vi "Sistema_2.vi"() -> ()   [LabVIEW 2017]
uses:
  <vilib>/Motion/Express/_s/nimc.ex.write.writeSetpoint.axis.vi
  <vilib>/Motion/Express/_s/nimc.fb.straightLineMove.startStraightLineMove.axis.modeAbsolute.0.vi
  <vilib>/Motion/Express/_s/nimc.fb.arcMove.startArcMove.coordinate.modeCircular.0.vi
  <vilib>/Motion/Express/_s/nimc.ex.read.readExecutionData.axis.vi
  <vilib>/Motion/BlockNode/FB.NIMotion.xnode
panel:
  in  "Array 2":T1(array[cluster])
  in  "Velocidad":dbl=10.0 format="%#_13g"
  out "x > y?":bool=TRUE
  out "done":bool=TRUE
  in  "Posición Inicial":cluster{"X":dbl, "Y":dbl, "Z":dbl}
  out "Paso":i32=69
  in  "Stop Button":bool
  out "EY":dbl(slide) scale=0.0..10.0
  out "EX":dbl(slide)=23.0 scale=0.0..10.0
  out "XY Graph":cluster{dbl[], dbl[]}(graph)={[0.0, 0.426423996, 1.426315789, 2.4263157890000002, 2.999891794, 3.0, 2.997709298, 2.215789474, 1.218080176, 1.0, 1.0, 1.0, 1.0, 1.0, 1.0, 0.45789473700000005, -0.0, -0.0, -0.0, -0.0, -0.0, -0.0, -0.0, 0.005048895, 0.32563547000000004, 1.194736842, 2.194736842, 2.894736842, 3.894736842, 4.894736842, 5.894736842, 6.727090094, 6.998255176, 7.0, 7.0, 7.0, 7.0, 7.0, 7.0, 7.0, 6.557894737, 6.0, 6.0, 6.0, 6.0, 6.0, 6.0, 5.557894737, 5.0, 5.0, 5.0, 5.0, 5.0, 5.0, 5.0, 4.157894737, 4.0, 4.0, 4.0, 4.0, 4.0, 4.0, 4.0, 4.048989208, 4.516094471, 5.436842105, 6.436842105, 7.436842105, 8.436842105, 9.436842105, 10.436842105, 11.387852897, 11.920747634, 12.0, 12.0, 11.916385042, 10.936842105, 10.5, 10.5, 10.5, 10.5, 10.5, 11.063157895, 11.979542936, 12.0, 12.0, 11.995418596, 11.529091619999999, 10.531578947, 9.531578947, 8.532151623, 8.002487327, 8.0, 8.0, 8.763157895, 9.5, 9.5, 9.5, 9.5, 9.5, 9.136842105, 8.066802093, 8.0, 8.0, 8.055501693, 8.564273623, 9.515789474, 10.515789474, 11.515789474, 12.515789474, 13.515789474, 14.514486319, 15.27534626, 15.499221793, 15.990506967, 16.0, 16.0, 15.584, 15.057894737, 14.5, 14.0, 14.116, 14.607617729, 15.601898554, 15.999811191, 16.0, 15.75, 15.105263158, 14.105263158, 13.5, 13.0, 13.0, 13.0, 13.0, 13.509032779, 14.486361958, 14.990506967, 15.0, 14.5, 13.836842105, 13.001629181, 13.0, 13.092082839, 13.707674496, 14.694736842, 15.694736842, 16.694736842, 17.694736842, 18.694736842, 19.602654003, 19.987062346000002, 20.0, 20.0, 20.0, 20.111486611, 21.084210526, 21.972723915, 22.0, 22.0, 21.415789474, 20.415789474, 20.0, 20.0, 20.111486611, 21.084210526, 21.972723915, 22.0, 22.0, 21.573576004, 20.573684211, 19.573684211, 19.0, 19.0, 19.0, 19.0, 19.0, 19.0, 19.0, 19.0, 19.167646748, 19.896481666, 20.894736842, 21.894736842, 22.894736842, 23.894736842, 24.994549846, 25.780379567, 25.999747518, 26.0, 26.0, 25.315789474, 24.218080176, 24.0, 24.0, 24.284282664, 25.284210526, 25.999927862, 26.0, 25.997709298, 25.215789474, 24.218080176, 24.0, 24.0, 24.284282664, 25.284210526, 25.999927862, 26.0, 25.99898191, 25.373684211, 24.373684211, 23.3747023, 23.0, 23.0, 23.0, 23.0, 23.0, 23.0, 23.0], [0.0, 0.0, 0.0, 0.0, 0.0, 0.5421052630000001, 1.0, 1.0, 1.0, 1.004581404, 1.568565328, 2.568421053, 3.568421053, 4.563839648, 4.999855725, 5.0, 5.0, 4.721283472, 3.789473684, 2.789473684, 1.6894736840000002, 0.689840197, 0.039900739000000005, 0.0, 0.0, 0.0, 0.0, 0.0, 0.0, 0.0, 0.0, 0.0, 0.0, 0.045163897, 0.71070666, 1.7105263160000002, 2.710526316, 3.610526316, 4.587072946, 4.997899781, 5.0, 5.0, 4.621142376, 3.631578947, 2.631578947, 1.532151623, 1.002487327, 1.0, 1.0, 1.3788576240000001, 2.268421053, 2.968421053, 3.868421053, 4.801204409, 5.0, 5.0, 4.97654663, 4.28929334, 3.289473684, 2.289473684, 1.289473684, 0.334637581, 0.000180344, 0.0, 0.0, 0.0, 0.0, 0.0, 0.0, 0.0, 0.0, 0.0, 0.0, 0.0, 0.742105263, 1.0, 1.0, 1.0, 1.5263157889999999, 2.526315789, 3.526315789, 4.0, 4.0, 4.0, 4.442105263, 5.0, 5.0, 5.0, 5.0, 5.0, 5.0, 5.0, 4.557894737, 4.0, 4.0, 4.0, 3.670425848, 2.6736842110000003, 1.673684211, 1.003258362, 1.0, 1.0, 0.657894737, -0.0, -0.0, -0.0, -0.0, -0.0, -0.0, -0.0, -0.0, -0.0, -0.0, -0.0, 0.490506967, 0.963157895, 1.933197907, 2.416, 2.5, 2.5, 3.025493033, 3.616, 4.0, 4.0, 4.249811191, 4.75, 5.0, 5.0, 5.0, 5.0, 4.5, 3.9157894740000003, 2.9157894740000003, 2.5, 2.0, 2.0, 1.509493033, 1.0, 0.5, 0.5, 0.5, 0.0, 0.0, 0.0, 0.0, 0.0, 0.0, 0.0, 0.0, 0.0, 0.0, 0.05435941800000001, 0.984210526, 1.929851108, 2.0, 2.0, 2.0, 2.342105263, 3.0, 3.0, 3.0, 3.0, 3.842105263, 4.0, 4.0, 4.0, 4.342105263, 5.0, 5.0, 5.0, 5.0, 5.0, 4.839704524, 3.989473684, 2.989473684, 1.989473684, 0.989473684, 0.14976916, -0.0, -0.0, -0.0, -0.0, -0.0, -0.0, -0.0, -0.0, -0.0, -0.0, 0.442105263, 1.0, 1.0, 1.0, 1.055743306, 1.986361958, 2.0, 2.0, 2.0, 2.542105263, 3.0, 3.0, 3.0, 3.055743306, 3.986361958, 4.0, 4.0, 4.0, 4.542105263, 5.0, 5.0, 5.0, 5.0, 5.0, 4.721283472, 3.789473684, 2.789473684, 1.789473684, 0.7894736840000001, 0.068190212]}
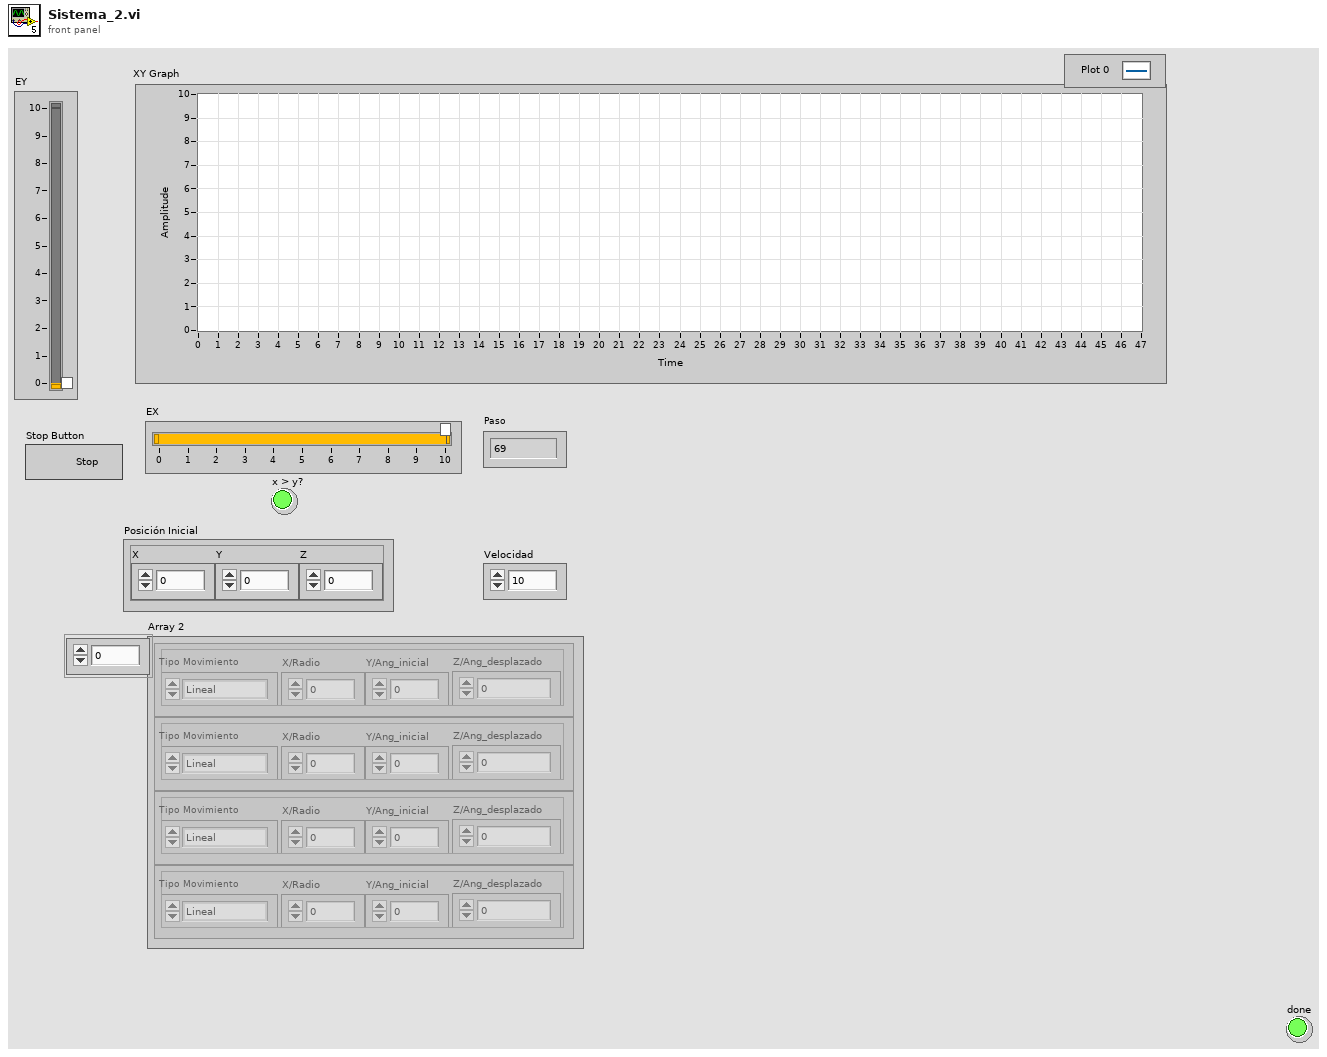
[diagram p1: front panel]
types:
  T1 = cluster{"Tipo Movimiento":enum16{"Lineal", "Circular"}, "X/Radio":dbl, "Y/Ang_inicial":dbl, "Z/Ang_desplazado":dbl}[]
  T2 = cluster{"Tipo Movimiento":enum16{"Lineal", "Circular"}, "X":dbl, "Y":dbl}[]
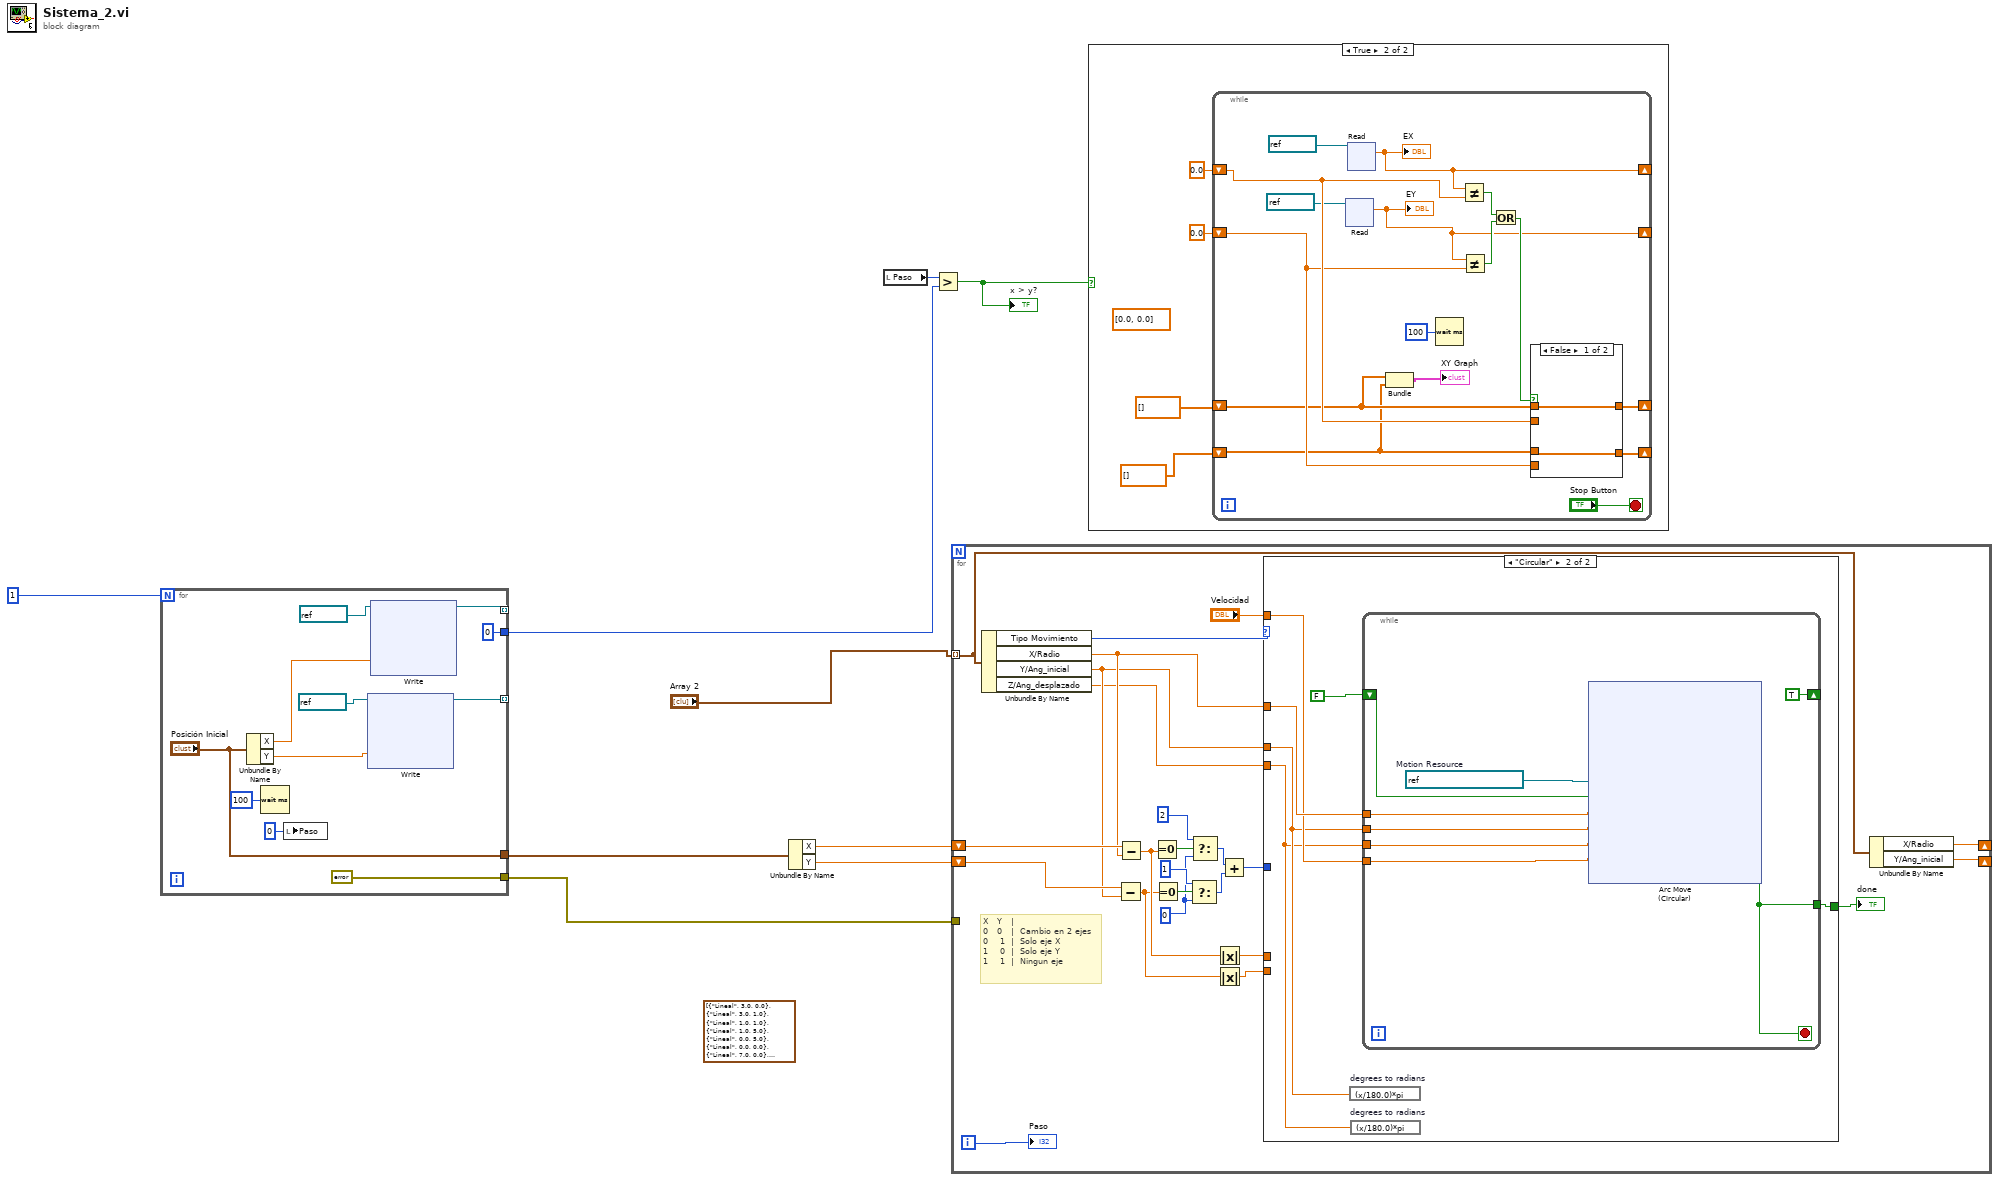
[diagram p0: block diagram]
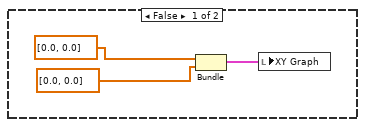
[diagram p2: hidden frame]
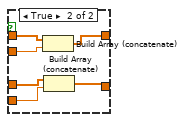
[diagram p3: hidden frame]
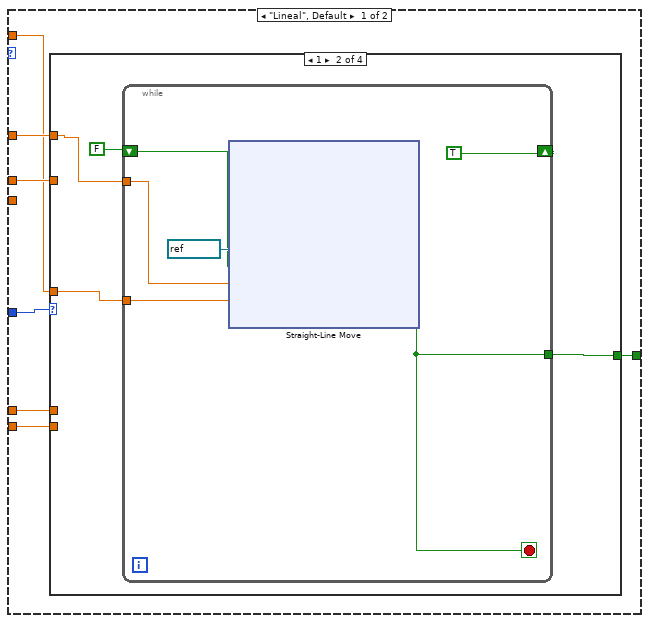
[diagram p4: hidden frame]
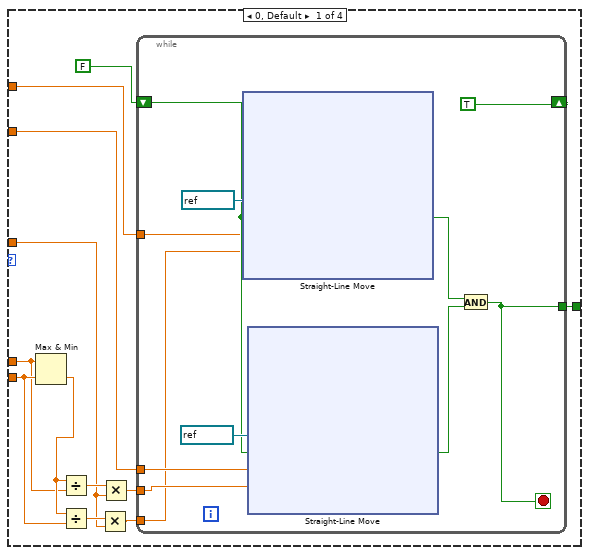
[diagram p5: hidden frame]
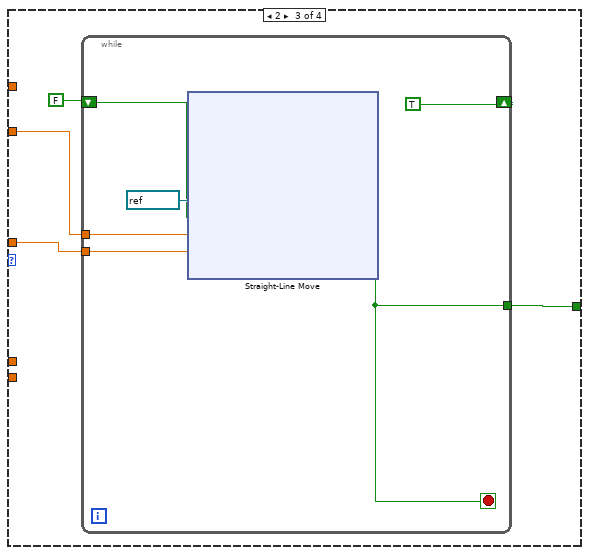
[diagram p6: hidden frame]
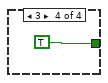
[diagram p7: hidden frame]
diagram:
  (unwired) T2 [{"Tipo Movimiento"=enum."Lineal", "X"=3.0, "Y"=0.0}, {"Tipo Movimiento"=enum."Lineal", "X"=3.0, "Y"=1.0}, {"Tipo Movimiento"=enum."Lineal", "X"=1.0, "Y"=1.0}, {"Tipo Movimiento"=enum."Lineal", "X"=1.0, "Y"=5.0}, {"Tipo Movimiento"=enum."Lineal", "X"=0.0, "Y"=5.0}, {"Tipo Movimiento"=enum."Lineal", "X"=0.0, "Y"=0.0}, {"Tipo Movimiento"=enum."Lineal", "X"=7.0, "Y"=0.0}, {"Tipo Movimiento"=enum."Lineal", "X"=7.0, "Y"=5.0}, {"Tipo Movimiento"=enum."Lineal", "X"=6.0, "Y"=5.0}, {"Tipo Movimiento"=enum."Lineal", "X"=6.0, "Y"=1.0}, {"Tipo Movimiento"=enum."Lineal", "X"=5.0, "Y"=1.0}, {"Tipo Movimiento"=enum."Lineal", "X"=5.0, "Y"=5.0}, {"Tipo Movimiento"=enum."Lineal", "X"=4.0, "Y"=5.0}, {"Tipo Movimiento"=enum."Lineal", "X"=4.0, "Y"=0.0}, {"Tipo Movimiento"=enum."Lineal", "X"=12.0, "Y"=0.0}, {"Tipo Movimiento"=enum."Lineal", "X"=12.0, "Y"=1.0}, {"Tipo Movimiento"=enum."Lineal", "X"=10.5, "Y"=1.0}, {"Tipo Movimiento"=enum."Lineal", "X"=10.5, "Y"=4.0}, {"Tipo Movimiento"=enum."Lineal", "X"=12.0, "Y"=4.0}, {"Tipo Movimiento"=enum."Lineal", "X"=12.0, "Y"=5.0}, {"Tipo Movimiento"=enum."Lineal", "X"=8.0, "Y"=5.0}, {"Tipo Movimiento"=enum."Lineal", "X"=8.0, "Y"=4.0}, {"Tipo Movimiento"=enum."Lineal", "X"=9.5, "Y"=4.0}, {"Tipo Movimiento"=enum."Lineal", "X"=9.5, "Y"=1.0}, {"Tipo Movimiento"=enum."Lineal", "X"=8.0, "Y"=1.0}, {"Tipo Movimiento"=enum."Lineal", "X"=8.0, "Y"=0.0}, {"Tipo Movimiento"=enum."Lineal", "X"=15.5, "Y"=0.0}, {"Tipo Movimiento"=enum."Lineal", "X"=16.0, "Y"=0.5}, {"Tipo Movimiento"=enum."Lineal", "X"=16.0, "Y"=2.0}, {"Tipo Movimiento"=enum."Lineal", "X"=15.5, "Y"=2.5}, {"Tipo Movimiento"=enum."Lineal", "X"=14.5, "Y"=2.5}, {"Tipo Movimiento"=enum."Lineal", "X"=14.0, "Y"=3.0}, {"Tipo Movimiento"=enum."Lineal", "X"=14.0, "Y"=3.5}, {"Tipo Movimiento"=enum."Lineal", "X"=14.5, "Y"=4.0}, {"Tipo Movimiento"=enum."Lineal", "X"=15.75, "Y"=4.0}, {"Tipo Movimiento"=enum."Lineal", "X"=16.0, "Y"=4.25}, {"Tipo Movimiento"=enum."Lineal", "X"=16.0, "Y"=4.75}, {"Tipo Movimiento"=enum."Lineal", "X"=15.75, "Y"=5.0}, {"Tipo Movimiento"=enum."Lineal", "X"=13.5, "Y"=5.0}, {"Tipo Movimiento"=enum."Lineal", "X"=13.0, "Y"=4.5}, {"Tipo Movimiento"=enum."Lineal", "X"=13.0, "Y"=2.5}, {"Tipo Movimiento"=enum."Lineal", "X"=13.5, "Y"=2.0}, {"Tipo Movimiento"=enum."Lineal", "X"=14.5, "Y"=2.0}, {"Tipo Movimiento"=enum."Lineal", "X"=15.0, "Y"=1.5}, {"Tipo Movimiento"=enum."Lineal", "X"=15.0, "Y"=1.0}, {"Tipo Movimiento"=enum."Lineal", "X"=14.5, "Y"=0.5}, {"Tipo Movimiento"=enum."Lineal", "X"=13.0, "Y"=0.5}, {"Tipo Movimiento"=enum."Lineal", "X"=13.0, "Y"=0.0}, {"Tipo Movimiento"=enum."Lineal", "X"=20.0, "Y"=0.0}, {"Tipo Movimiento"=enum."Lineal", "X"=20.0, "Y"=2.0}, {"Tipo Movimiento"=enum."Lineal", "X"=22.0, "Y"=2.0}, {"Tipo Movimiento"=enum."Lineal", "X"=22.0, "Y"=3.0}, {"Tipo Movimiento"=enum."Lineal", "X"=20.0, "Y"=3.0}, {"Tipo Movimiento"=enum."Lineal", "X"=20.0, "Y"=4.0}, {"Tipo Movimiento"=enum."Lineal", "X"=22.0, "Y"=4.0}, {"Tipo Movimiento"=enum."Lineal", "X"=22.0, "Y"=5.0}, {"Tipo Movimiento"=enum."Lineal", "X"=19.0, "Y"=5.0}, {"Tipo Movimiento"=enum."Lineal", "X"=19.0, "Y"=0.0}, {"Tipo Movimiento"=enum."Lineal", "X"=26.0, "Y"=0.0}, {"Tipo Movimiento"=enum."Lineal", "X"=26.0, "Y"=1.0}, {"Tipo Movimiento"=enum."Lineal", "X"=24.0, "Y"=1.0}, {"Tipo Movimiento"=enum."Lineal", "X"=24.0, "Y"=2.0}, {"Tipo Movimiento"=enum."Lineal", "X"=26.0, "Y"=2.0}, {"Tipo Movimiento"=enum."Lineal", "X"=26.0, "Y"=3.0}, {"Tipo Movimiento"=enum."Lineal", "X"=24.0, "Y"=3.0}, {"Tipo Movimiento"=enum."Lineal", "X"=24.0, "Y"=4.0}, {"Tipo Movimiento"=enum."Lineal", "X"=26.0, "Y"=4.0}, {"Tipo Movimiento"=enum."Lineal", "X"=26.0, "Y"=5.0}, {"Tipo Movimiento"=enum."Lineal", "X"=23.0, "Y"=5.0}, {"Tipo Movimiento"=enum."Lineal", "X"=23.0, "Y"=0.0}, {"Tipo Movimiento"=enum."Lineal", "X"=27.5, "Y"=0.0}, {"Tipo Movimiento"=enum."Lineal", "X"=27.5, "Y"=2.0}, {"Tipo Movimiento"=enum."Lineal", "X"=28.0, "Y"=2.0}, {"Tipo Movimiento"=enum."Lineal", "X"=29.0, "Y"=0.0}, {"Tipo Movimiento"=enum."Lineal", "X"=30.0, "Y"=0.0}, {"Tipo Movimiento"=enum."Lineal", "X"=30.0, "Y"=1.0}, {"Tipo Movimiento"=enum."Lineal", "X"=29.0, "Y"=2.5}] ("Array 2")
  n1 = for {
    N: 1 -> [_]
    tunnel: [errorcluster {"status"=FALSE, "code"=0, "source"=""} ("error in")] -> w2
    tunnel: ["Posición Inicial"] -> w8
    tunnel: [w16] -> _ mode=indexing
    tunnel: [w15] -> _ mode=indexing
    tunnel: [0 ("y")] -> w3
    n2 = Unbundle By Name("Posición Inicial") -> ("X"=w10:dbl, "Y"=w14:dbl)
    n3 = Wait (ms)(milliseconds to wait=u32 100) -> ()  [unwired: 1 out]
    n4 = local write "Paso"(0 ("Paso")) -> ()
    n5 = xnode ("Write")("position setpoint"=w14, "resource"=refnum<k21> "Eje Y" ("Motion Resource")) -> ("resource out"=w16:refnum<k21>)  [unwired: 1 in, 1 out]
    n6 = xnode ("Write")("position setpoint"=w10, "resource"=refnum<k21> "Eje X" ("Motion Resource")) -> ("resource out"=w15:refnum<k21>)  [unwired: 1 in, 1 out]
  }
  n7 = Unbundle By Name(w8) -> ("X"=w7:dbl, "Y"=w6:dbl)
  n8 = local read "Paso"() -> (w5:i32)
  n9 = Greater?(x=w5, y=w3) -> (0:w4:bool)
  "x > y?" <- w4
  n10 = for {
    tunnel: "Array 2" -> [w52] mode=indexing
    tunnel: w2 -> [_]
    shift-right: [w50] -> _
    shift-left: w6 -> [w47]
    shift-right: [w51] -> _
    shift-left: w7 -> [w49]
    i -> [w53]
    w41 = 0 ("f")
    # "X   Y   |\n0   0   |  Cambio en 2 ejes\n0    1  |  Solo eje X\n1    0  |  Solo eje Y\n1    1  |  Ningun eje"
    n11 = Unbundle By Name(w52) -> ("Tipo Movimiento"=w54:enum16{"Lineal", "Circular"}, "X/Radio"=w48:dbl, "Y/Ang_inicial"=w46:dbl, "Z/Ang_desplazado"=w31:dbl)
    n12 = Subtract(x=w47, y=w46) -> (x-y=w34:dbl)
    n13 = Subtract(x=w49, y=w48) -> (x-y=w35:dbl)
    n14 = Equal To 0?(x=w35) -> (x = 0?=w45:bool)
    n15 = Equal To 0?(x=w34) -> (x = 0?=w43:bool)
    n16 = Select(t=1, s=w43, f=w41) -> (s? t:f=w39:i32)
    n17 = Select(t=2, s=w45, f=w41) -> (s? t:f=w40:i32)
    n18 = Absolute Value(x=w35) -> (abs(x)=w36:dbl)
    n19 = Absolute Value(x=w34) -> (abs(x)=w33:dbl)
    n20 = Add(x=w40, y=w39) -> (x+y=w38:i32)
    n21 = case shown="\"Circular\"" w54 {
      tunnel: w48 -> [w59 w179]
      tunnel: w46 -> [w58 w175]
      tunnel: w38 -> [w61 _]
      tunnel: [w60 w176] -> w37
      tunnel: w33 -> [w57 _]
      tunnel: w36 -> [w56 _]
      tunnel: "Velocidad" -> [w55 w178]
      tunnel: w31 -> [_ w174]
      frame "Lineal", Default {
        n22 = case shown="1" w61 {
          tunnel: [w72 w121 w148 TRUE] -> w60
          tunnel: w55 -> [w65 w120 w147 _]
          tunnel: w59 -> [w71 w119 _ _]
          tunnel: w58 -> [w70 _ w146 _]
          tunnel: w57 -> [w63 _ _ _]
          tunnel: w56 -> [w62 _ _ _]
          frame 0, Default {
            n23 = Max & Min(x=w62, y=w63) -> (min(x,y)=w64:dbl)  [unwired: 1 out]
            n24 = Divide(x=w64, y=w62) -> (x/y=w67:dbl)
            n25 = Divide(x=w64, y=w63) -> (x/y=w66:dbl)
            n26 = Multiply(x=w66, y=w65) -> (x*y=w69:dbl)
            n27 = Multiply(x=w67, y=w65) -> (x*y=w68:dbl)
            n28 = while {
              shift-right: [TRUE] -> _
              shift-left: FALSE -> [w81]
              tunnel: [w78] -> w72
              tunnel: w71 -> [w77]
              tunnel: w70 -> [w76]
              tunnel: w69 -> [w74]
              tunnel: w68 -> [w75]
              stop <- w78 stop-if-true
              n29 = xnode "Straight-Line Move"("resource"=refnum<k21> "Eje X" ("Motion Resource"), "execute"=w81, "position"=w77, "velocity"=w74) -> ("done"=w80:bool)  [unwired: 2 in, 2 out]
              n30 = xnode "Straight-Line Move"("resource"=refnum<k21> "Eje Y" ("Motion Resource"), "execute"=w81, "position"=w76, "velocity"=w75) -> ("done"=w79:bool)  [unwired: 2 in, 2 out]
              n31 = And(x=w80, y=w79) -> (x .and. y?=w78:bool)
            }
          }
          frame 1 {
            n32 = while {
              shift-right: [TRUE] -> _
              shift-left: FALSE -> [w126]
              tunnel: [w125] -> w121
              tunnel: w120 -> [w124]
              tunnel: w119 -> [w123]
              stop <- w125 stop-if-true
              n33 = xnode "Straight-Line Move"("resource"=refnum<k21> "Eje X" ("Motion Resource"), "execute"=w126, "position"=w123, "velocity"=w124) -> ("done"=w125:bool)  [unwired: 2 in, 2 out]
            }
          }
          frame 2 {
            n34 = while {
              shift-right: [TRUE] -> _
              shift-left: FALSE -> [w153]
              tunnel: [w152] -> w148
              tunnel: w147 -> [w151]
              tunnel: w146 -> [w150]
              stop <- w152 stop-if-true
              n35 = xnode "Straight-Line Move"("resource"=refnum<k21> "Eje Y" ("Motion Resource"), "execute"=w153, "position"=w150, "velocity"=w151) -> ("done"=w152:bool)  [unwired: 2 in, 2 out]
            }
          }
          frame 3 {
          }
        }
      }
      frame "Circular" {
        n36 = expression code="(x/180.0)*pi" "degrees to radians"(w175) -> ()  [unwired: 1 out]
        n37 = expression code="(x/180.0)*pi" "degrees to radians"(w174) -> ()  [unwired: 1 out]
        n38 = while {
          tunnel: w179 -> [w187]
          tunnel: w175 -> [w186]
          tunnel: w174 -> [w185]
          tunnel: w178 -> [w184]
          shift-right: [TRUE] -> _
          shift-left: FALSE -> [w183]
          tunnel: [w181] -> w176
          stop <- w181 stop-if-true
          w180 = refnum<k21> "Coordinate Space 1"  # Motion Resource
          n39 = xnode "Arc Move\n(Circular)"("resource"=w180, "execute"=w183, "radius"=w187, "start angle"=w186, "travel angle"=w185, "velocity"=w184) -> ("done"=w181:bool)  [unwired: 2 in, 2 out]
        }
      }
    }
    "done" <- w37
    n40 = Unbundle By Name(w52) -> ("X/Radio"=w51:dbl, "Y/Ang_inicial"=w50:dbl)
    "Paso" <- w53
  }
  n41 = case shown="True" w4 {
    frame False {
      n42 = Bundle(dbl[] [0.0, 0.0], dbl[] [0.0, 0.0]) -> (w207:cluster{dbl[], dbl[]})  [unwired: 1 in]
      n43 = local write "XY Graph"(w207) -> ()
    }
    frame True {
      (unwired) dbl[] [0.0, 0.0]
      n44 = while {
        shift-right: [w220] -> _
        shift-left: 0.0 ("position") -> [w226]
        shift-right: [w221] -> _
        shift-left: 0.0 ("position") -> [w225]
        shift-right: [w224] -> _
        shift-left: dbl[] [] -> [w217]
        shift-right: [w223] -> _
        shift-left: dbl[] [] -> [w218]
        stop <- "Stop Button" stop-if-true
        n45 = xnode "Read"("resource"=refnum<k21> "Eje Y" ("Motion Resource")) -> ("position"=w221:dbl)  [unwired: 1 in, 6 out]
        "EY" <- w221
        n46 = xnode "Read"("resource"=refnum<k21> "Eje X" ("Motion Resource")) -> ("position"=w220:dbl)  [unwired: 1 in, 6 out]
        "EX" <- w220
        n47 = Bundle(w218, w217) -> (→"XY Graph":cluster{dbl[], dbl[]})  [unwired: 1 in]
        n48 = Wait (ms)(milliseconds to wait=u32 100) -> ()  [unwired: 1 out]
        n49 = Not Equal?(x=w220, y=w226) -> (x != y?=w229:bool)
        n50 = Not Equal?(x=w221, y=w225) -> (x != y?=w228:bool)
        n51 = Or(x=w229, y=w228) -> (x .or. y?=w227:bool)
        n52 = case shown="False" w227 {
          tunnel: w218 -> [w231 w237]
          tunnel: w217 -> [w230 w234]
          tunnel: w226 -> [_ w236]
          tunnel: w225 -> [_ w233]
          tunnel: [w230 w232] -> w224
          tunnel: [w231 w235] -> w223
          frame False {
          }
          frame True {
            n53 = Build Array (concatenate)(w237, w236) -> (w235:dbl[])
            n54 = Build Array (concatenate)(w234, w233) -> (w232:dbl[])
          }
        }
      }
    }
  }
